vi "PXI-Compute Skip Samples.vi"(0 "AO Tasks":T1[](array[typedef]), 5 "AI Tasks":T2[](array[typedef]), 7 "AO Sample Rate":dbl, 9 "AI Sample Rate":dbl, 11 "error in (no error)":errorcluster) -> (8 "Skip Samples":i32, 15 "error out":errorcluster)   [LabVIEW 2020]
doc: "Determines the number of AI samples to skip in order to register AO and AI (accounting for the latencies of the 24-bit boards)."
uses:
  AIDI/Typedefs/AIDI-Task Specification.ctl
  AODO/Typedefs/AODO-Task Specification.ctl
panel:
  out "Any 16-bit AI?":bool
  out "Any 16-bit AO?":bool
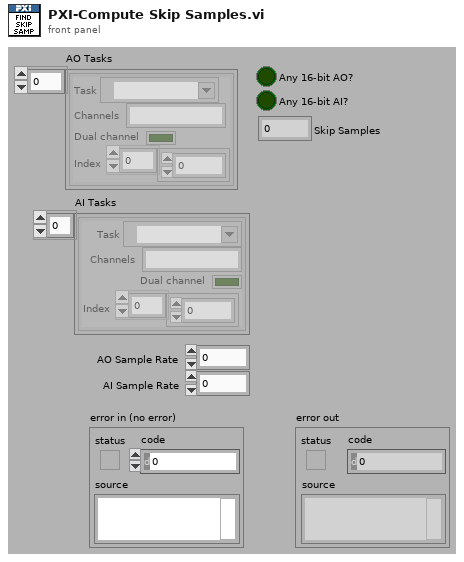
[diagram p1: front panel]
types:
  T1 = typedef "AODO-Task Specification.ctl" = cluster{"Task":refnum<k21>, "Channels":string, "Dual channel":bool, "Index":i32[]}
  T2 = typedef "AIDI-Task Specification.ctl" = cluster{"Task":refnum<k21>, "Channels":string, "Dual channel":bool, "Index":i32[]}
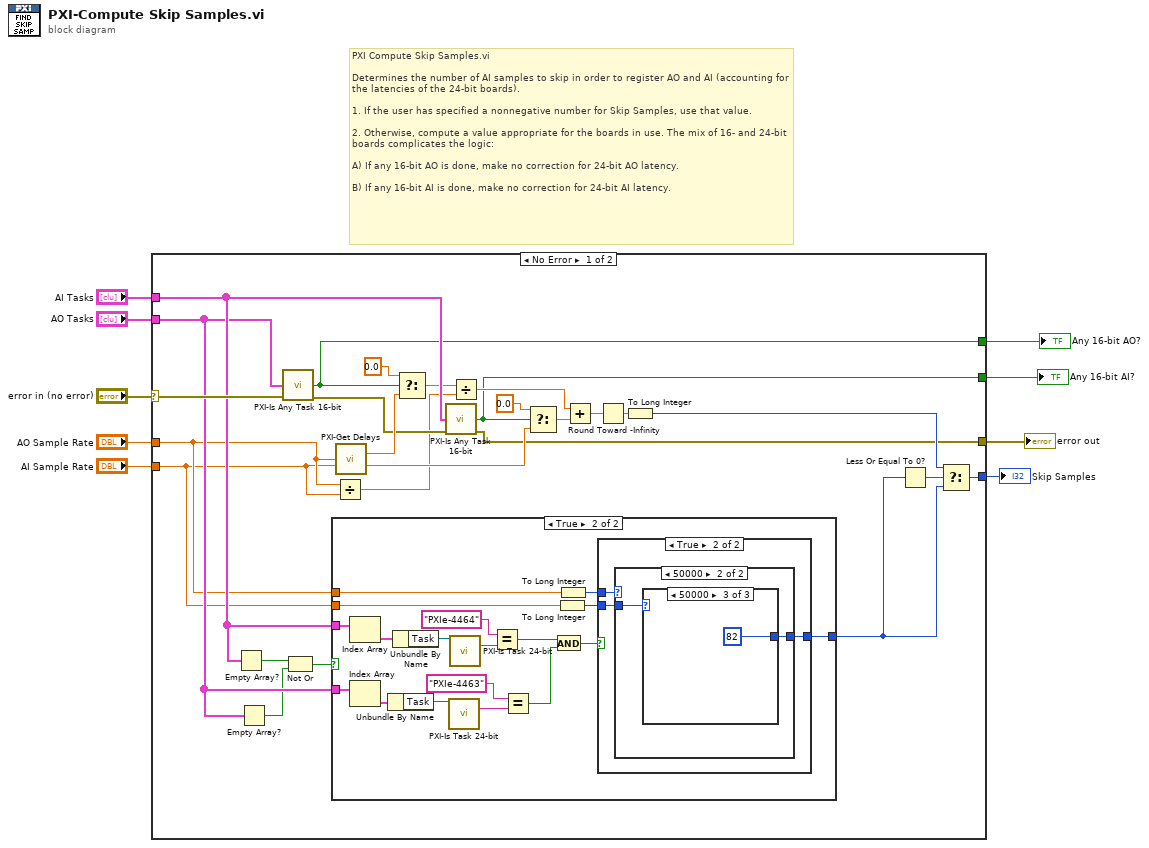
[diagram p0: block diagram]
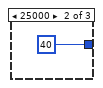
[diagram p6: hidden frame]
diagram:
  # "PXI Compute Skip Samples.vi\n\nDetermines the number of AI samples to skip in order to register AO and AI (accounting for the latencies of the 24-bit boards). \n\n1. If the user has specified a nonnegative number for Skip Samples, use that value. \n\n2. Otherwise, compute a value appropriate for the boards in use. The mix of 16- and 24-bit boards complicates the logic:\n\nA) If any 16-bit AO is done, make no correction for 24-bit AO latency.\n\nB) If any 16-bit AI is done, make no correction for 24-bit AI latency."
  n1 = case shown="No Error" "error in (no error)" {
    selector: "error in (no error)" -> [w35 w61]
    tunnel: "AI Tasks" -> [w34 _]
    tunnel: "AO Tasks" -> [w33 _]
    tunnel: [w28 _] -> w6
    tunnel: "AO Sample Rate" -> [w25 _]
    tunnel: "AI Sample Rate" -> [w24 _]
    tunnel: [w12 _] -> w3
    tunnel: [w11 _] -> w2
    tunnel: [w10 w61] -> w1
    frame No Error {
      n2 = Empty Array?(array=w34) -> (empty?=w32:bool)
      n3 = Empty Array?(array=w33) -> (empty?=w31:bool)
      n4 = call "PXI-Is Any Task 16-bit.vi"("Task Array"=w33, "error in (no error)"=w35) -> ("Any 16-bit task?"=w11:bool, "error out"=w19:errorcluster)  [unwired: 12 in]
      n5 = Not Or(1:w31, 2:w32) -> (0:w30:bool)
      n6 = case shown="True" w30 {
        tunnel: w34 -> [_ w48]
        tunnel: w33 -> [_ w47]
        tunnel: w25 -> [_ w43]
        tunnel: w24 -> [_ w41]
        tunnel: [_ w36] -> w27
        frame False {
        }
        frame True {
          n7 = Index Array(array=w48) -> (element=w53:T2)  [unwired: 1 in]
          n8 = Index Array(array=w47) -> (element=w52:T1)  [unwired: 1 in]
          n9 = Unbundle By Name(w52) -> ("Task"=w49:refnum<k21>)
          n10 = Unbundle By Name(w53) -> ("Task"=w51:refnum<k21>)
          n11 = call "PXI-Is Task 24-bit.vi"("task"=w49) -> ("Product Type"=w37:string)  [unwired: 9 in, 5 out]
          n12 = call "PXI-Is Task 24-bit.vi"("task"=w51) -> ("Product Type"=w38:string)  [unwired: 9 in, 5 out]
          n13 = Equal?(x="PXIe-4464", y=w38) -> (x = y?=w45:bool)
          n14 = Equal?(x="PXIe-4463", y=w37) -> (x = y?=w44:bool)
          n15 = And(x=w45, y=w44) -> (x .and. y?=w39:bool)
          n16 = To Long Integer(number=w41) -> (32bit integer=w40:i32)
          n17 = To Long Integer(number=w43) -> (32bit integer=w42:i32)
          n18 = case shown="True" w39 {
            tunnel: w42 -> [_ w56]
            tunnel: w40 -> [_ w55]
            tunnel: [_ w54] -> w36
            frame False {
            }
            frame True {
              n19 = case shown="50000" w56 {
                tunnel: w55 -> [_ w58]
                tunnel: [_ w57] -> w54
                frame 0, Default {
                }
                frame 50000 {
                  n20 = case shown="50000" w58 {
                    tunnel: [_ 40 82] -> w57
                    frame 0, Default {
                    }
                    frame 25000 {
                    }
                    frame 50000 {
                    }
                  }
                }
              }
            }
          }
        }
      }
      n21 = Divide(x=w25, y=w24) -> (x/y=w13:dbl)
      n22 = call "PXI-Get Delays.vi"("AO Rate (Samples/s)"=w25, "AI Rate (Samples/s)"=w24) -> ("AO delay (samples)"=w20:dbl, "AI delay (samples)"=w18:dbl)  [unwired: 12 in]
      n23 = Select(t=0.0 ("f"), s=w11, f=w20) -> (s? t:f=w15:dbl)
      n24 = call "PXI-Is Any Task 16-bit.vi"("Task Array"=w34, "error in (no error)"=w19) -> ("Any 16-bit task?"=w12:bool, "error out"=w10:errorcluster)  [unwired: 12 in]
      n25 = Divide(x=w15, y=w13) -> (x/y=w14:dbl)
      n26 = Select(t=0.0, s=w12, f=w18) -> (s? t:f=w16:dbl)
      n27 = Add(x=w14, y=w16) -> (x+y=w22:dbl)
      n28 = Round Toward -Infinity(1:w22) -> (0:w23:dbl)
      n29 = To Long Integer(number=w23) -> (32bit integer=w29:i32)
      n30 = Less Or Equal To 0?(x=w27) -> (x <= 0?=w26:bool)
      n31 = Select(t=w29, s=w26, f=w27) -> (s? t:f=w28:i32)
    }
    frame Error {
    }
  }
  "Skip Samples" <- w6
  "Any 16-bit AO?" <- w2
  "Any 16-bit AI?" <- w3
  "error out" <- w1
